vi "Pulse Divider.vi"() -> ()   [LabVIEW 2011]
uses:
  <vilib>/DAQmx/create/channels.llb/DAQmx Create Channel (CO-Pulse Generation-Ticks).vi
  <vilib>/DAQmx/configure/timing.llb/DAQmx Timing (Implicit).vi
panel:
  in  "Stop":bool
  in  "counter":tag="Dev1/ctr7"
  in  "Divide Factor":dbl=32000.0
  in  "source of ticks":tag="/4498_1/ai/SampleClock"
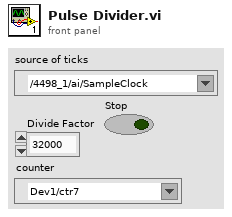
[diagram p1: front panel]
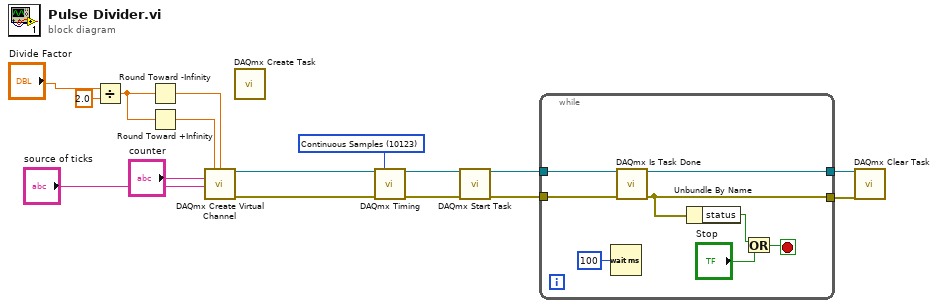
[diagram p0: block diagram]
diagram:
  w7 = 10123 items=["Finite Samples"=10178, "Continuous Samples"=10123, "Hardware Timed Single Point"=12522] ("sample mode")
  n1 = Divide(x="Divide Factor", y=2.0) -> (x/y=w13:dbl)
  n2 = Round Toward -Infinity(1:w13) -> (0:w11:dbl)
  n3 = Round Toward +Infinity(x=w13) -> (ceil(x): smallest int >= x=w12:dbl)
  n4 = call-poly <vilib>:"DAQmx Create Virtual Channel.vi"("high ticks"=w12, "low ticks"=w11, "counter"="counter", "source of ticks"="source of ticks") -> ("task out"=w9:refnum<k21>, "error out"=w8:errorcluster)  [unwired: 10 in]
  n5 = call <vilib>:"DAQmx Create Task.vi"() -> ()  [unwired: 14 in, 2 out]
  n6 = call-poly <vilib>:"DAQmx Timing.vi"("task/channels in"=w9, "sample mode"=w7, "error in"=w8) -> ("task out"=w6:refnum<k21>, "error out"=w5:errorcluster)  [unwired: 11 in]
  n7 = call <vilib>:"DAQmx Start Task.vi"("task/channels in"=w6, "error in"=w5) -> ("task out"=w4:refnum<k21>, "error out"=w3:errorcluster)  [unwired: 12 in]
  n8 = while {
    tunnel: w4 -> [w24]
    tunnel: w3 -> [w23]
    tunnel: [w22] -> w1
    tunnel: [w17] -> w2
    stop <- w19 stop-if-true
    n9 = Wait (ms)(milliseconds to wait=u32 100) -> ()  [unwired: 1 out]
    n10 = call <vilib>:"DAQmx Is Task Done.vi"("task/channels in"=w24, "error in"=w23) -> ("task out"=w17:refnum<k21>, "error out"=w22:errorcluster)  [unwired: 11 in, 1 out]
    n11 = Unbundle By Name(w22) -> ("status"=w21:bool)
    n12 = Or(x=w21, y="Stop") -> (x .or. y?=w19:bool)
  }
  n13 = call <vilib>:"DAQmx Clear Task.vi"("task in"=w2, "error in"=w1) -> ()  [unwired: 13 in, 1 out]
